vi "ExecuteMenuItem.vi"(8 "error in (no error)":errorcluster caption="错误输入（无错误）", 10 "项标识符":string, 11 "listbox 输入":refnum<class "listbox.lvclass">) -> (0 "error out":errorcluster caption="错误输出", 3 "listbox 输出":refnum<class "listbox.lvclass">)   [LabVIEW 2016, in "listbox.lvclass"]
uses:
  listbox.lvclass
  listbox.lvclass/listbox.ctl
  LNK/Parent Class/Menu.lvclass
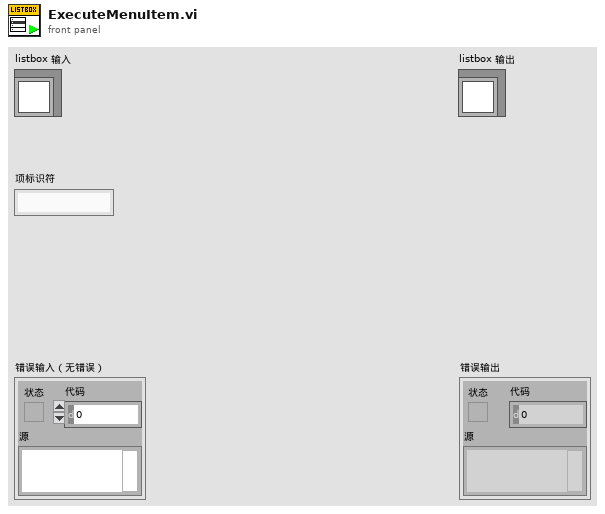
[diagram p1: front panel]
types:
  T1 = typedef "LVRowAndColumnTypeDef.ctl" = cluster{"Row":i32, "Column":i32}
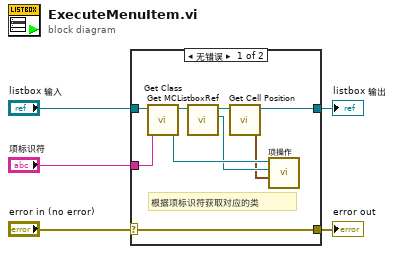
[diagram p0: block diagram]
diagram:
  n1 = case shown="无错误" "error in (no error)" {
    selector: "error in (no error)" -> [w13 w16]
    tunnel: [w13 w16] -> w4
    tunnel: [w7 w15] -> w2
    tunnel: "listbox 输入" -> [w14 w15]
    tunnel: "项标识符" -> [w11 _]
    frame No Error {
      # "根据项标识符获取对应的类"
      n2 = call "Get Class.vi"("listbox 输入"=w14, "项标识符"=w11) -> ("listbox 输出"=w12:refnum<class "listbox.lvclass">, "Menu.lvclass"=w10:refnum<class "Menu.lvclass">)  [unwired: 6 in, 1 out]
      n3 = call "Get MCListboxRef.vi"("listbox in"=w12) -> ("MCListboxRef"=w8:refnum<vi>, "listbox out"=w9:refnum<class "listbox.lvclass">)  [unwired: 9 in]
      n4 = call "Get Cell Position.vi"("listbox in"=w9) -> ("Cell Position"=w6:T1, "listbox out"=w7:refnum<class "listbox.lvclass">)  [unwired: 9 in]
      n5 = call-dynamic "项操作.vi"("Cell Position"=w6, "MCListbox引用句柄"=w8, "LNK 输入"=w10) -> ()  [unwired: 7 in, 2 out]
    }
    frame Error {
    }
  }
  "error out" <- w4
  "listbox 输出" <- w2
